vi "ELVIS III v1.0 DO Block Write.vi"(5 "Wait Until Done?":bool, 6 "DO FIFO Sample Rate (Hz)":dbl=1000.0 min=1000.0 max=8000000.0, 8 "error in (no error)":errorcluster, 9 "Data by Channel":bool[][](array[boolean]) caption="bool Value List", 10 "DO (N Samples) Channel List":T3, 11 "myRIO Ref In":T1) -> (0 "error out":errorcluster, 3 "myRIO Ref Out":T1)   [LabVIEW 2021]
uses:
  <vilib>/myRIO/Common/Instrument Driver Framework/myRIO v1.0/DO Block/typedefs/DO Block Channels List.ctl
  <vilib>/myRIO/Common/Instrument Driver Framework/myRIO v1.0/DO Block/typedefs/DO Block Channels Enum.ctl
  <vilib>/myRIO/Common/Instrument Driver Framework/Utilities/typedefs/myRIO v1.0 Reference.ctl
  <vilib>/myRIO/Common/Instrument Driver Framework/Utilities/typedefs/Generic FPGA Reference.ctl
  <vilib>/myRIO/Common/Instrument Driver Framework/ELVIS III v1.0/DO Block/typedefs/ELVIS III DO Block FPGA Reference.ctl
  <vilib>/myRIO/Common/Instrument Driver Framework/ELVIS III v1.0/DO Block/typedefs/ELVIS III DO Block Configuration.ctl
  <vilib>/myRIO/Common/Instrument Driver Framework/ELVIS III v1.0/DO Block/typedefs/ELVIS III DO Block Bank Data.ctl
  <vilib>/myRIO/Common/Instrument Driver Framework/myRIO v1.0/Resource Manager/vis/myRIO v1.0 Block Write Configuration.vi
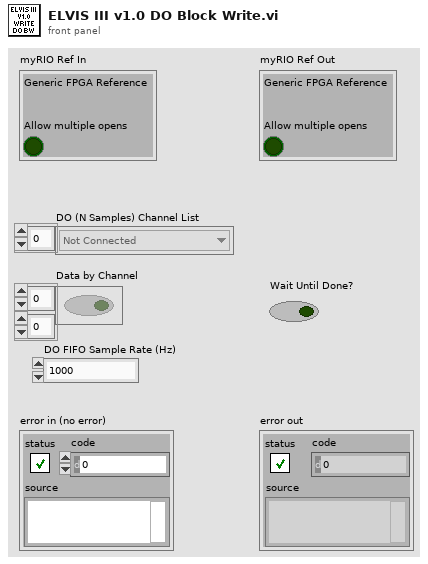
[diagram p1: front panel]
types:
  T1 = typedef "myRIO v1.0 Reference.ctl" = cluster{"Generic FPGA Reference":T2, "Allow multiple opens":bool}
  T2 = typedef "Generic FPGA Reference.ctl" = refnum<k20>
  T3 = typedef "DO Block Channels List.ctl" = T4[]
  T4 = typedef "DO Block Channels Enum.ctl" = enum16{"Not Connected", "A/DO0 (N Samples)", "A/DO1 (N Samples)", "A/DO2 (N Samples)", "A/DO3 (N Samples)", "A/DO4 (N Samples)", "A/DO5 (N Samples)", "A/DO6 (N Samples)", "A/DO7 (N Samples)", "A/DO8 (N Samples)", "A/DO9 (N Samples)", "A/DO10 (N Samples)", "A/DO11 (N Samples)", "A/DO12 (N Samples)", "A/DO13 (N Samples)", "A/DO14 (N Samples)", "A/DO15 (N Samples)", "A/DO16 (N Samples)", "A/DO17 (N Samples)", "A/DO18 (N Samples)", "A/DO19 (N Samples)", "B/DO0 (N Samples)", "B/DO1 (N Samples)", "B/DO2 (N Samples)", "B/DO3 (N Samples)", "B/DO4 (N Samples)", "B/DO5 (N Samples)", "B/DO6 (N Samples)", "B/DO7 (N Samples)", "B/DO8 (N Samples)", "B/DO9 (N Samples)", "B/DO10 (N Samples)", "B/DO11 (N Samples)", "B/DO12 (N Samples)", "B/DO13 (N Samples)", "B/DO14 (N Samples)", "B/DO15 (N Samples)", "B/DO16 (N Samples)", "B/DO17 (N Samples)", "B/DO18 (N Samples)", "B/DO19 (N Samples)"}
  T5 = typedef "ELVIS III DO Block FPGA Reference.ctl" = refnum<k20>
  T6 = typedef "ELVIS III DO Block Configuration.ctl" = cluster{"Wait Until Done?":bool, "DO FIFO Clock Divisor":u16, "Write Mode":u8, "DO (N Samples) Bank Data ":T7[]}
  T7 = typedef "ELVIS III DO Block Bank Data.ctl" = cluster{"Digital Data Reference":refnum<data-value>, "Channel  Bitmask":fxp<+,20,20>, "Semaphore":T8}
  T8 = typedef "Semaphore RefNum" = refnum<k1>
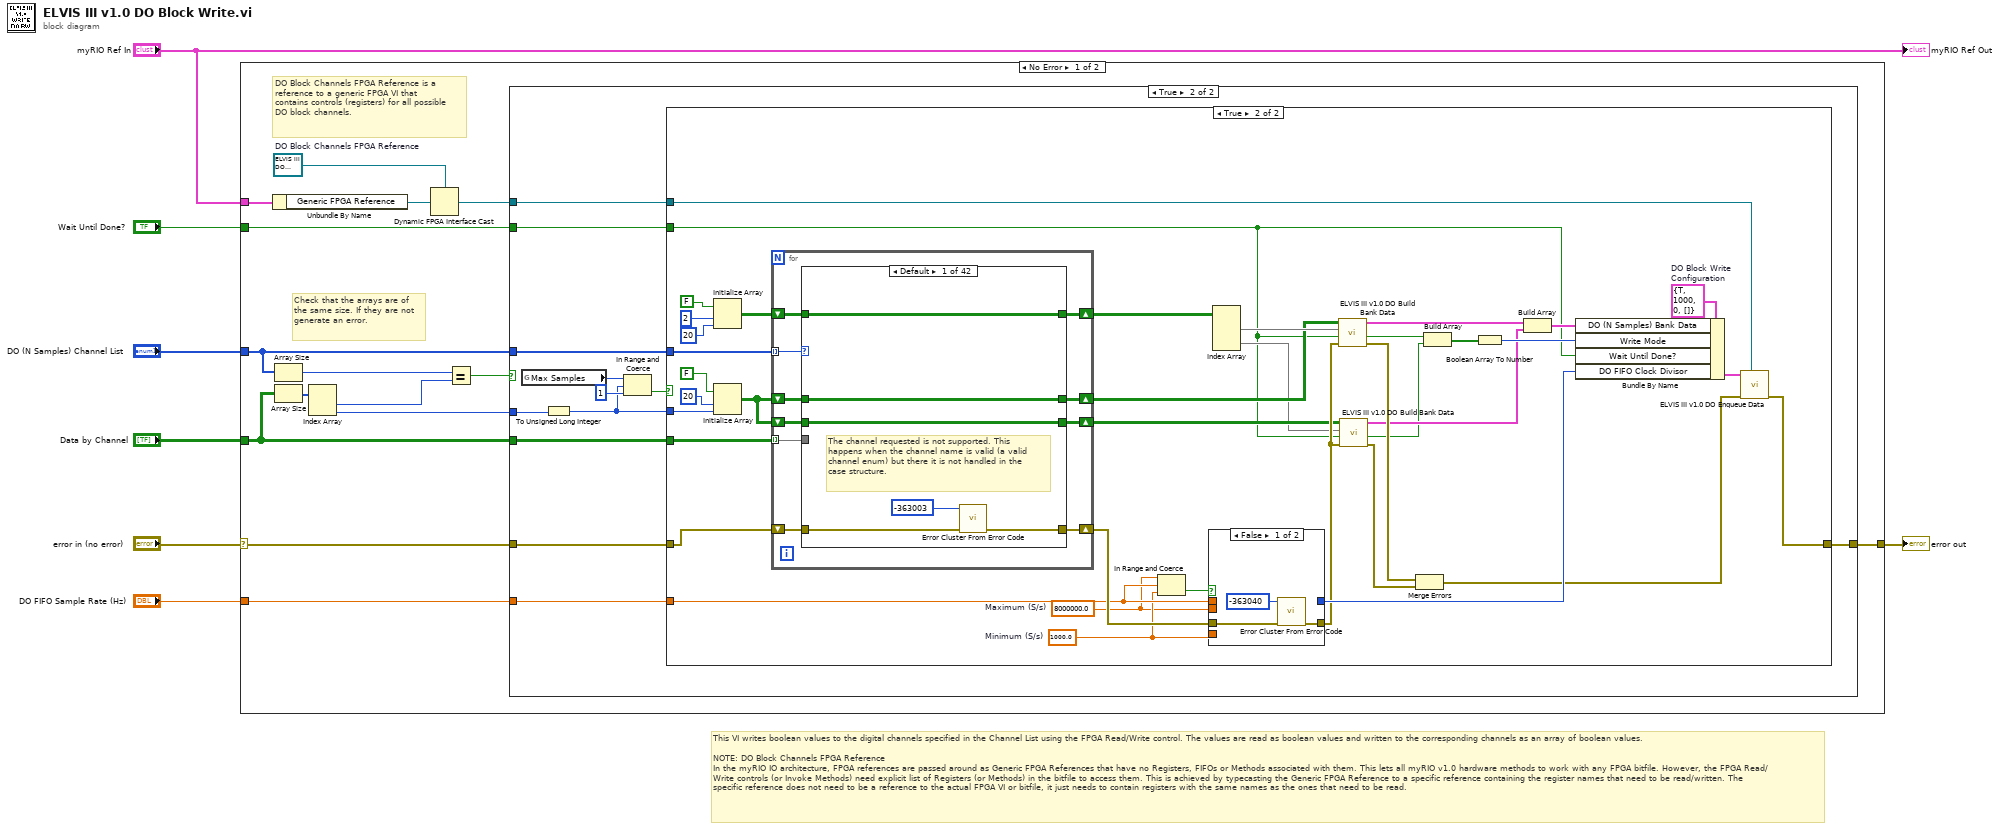
[diagram p0: block diagram]
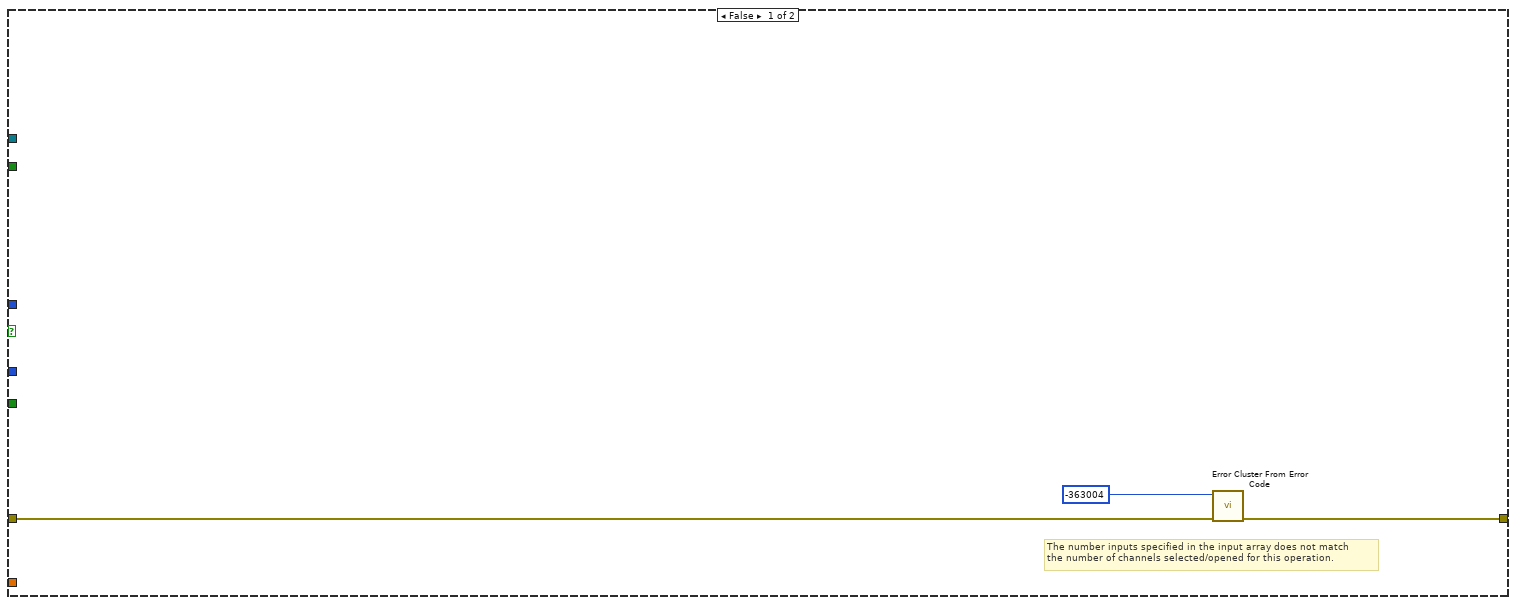
[diagram p2: hidden frame]
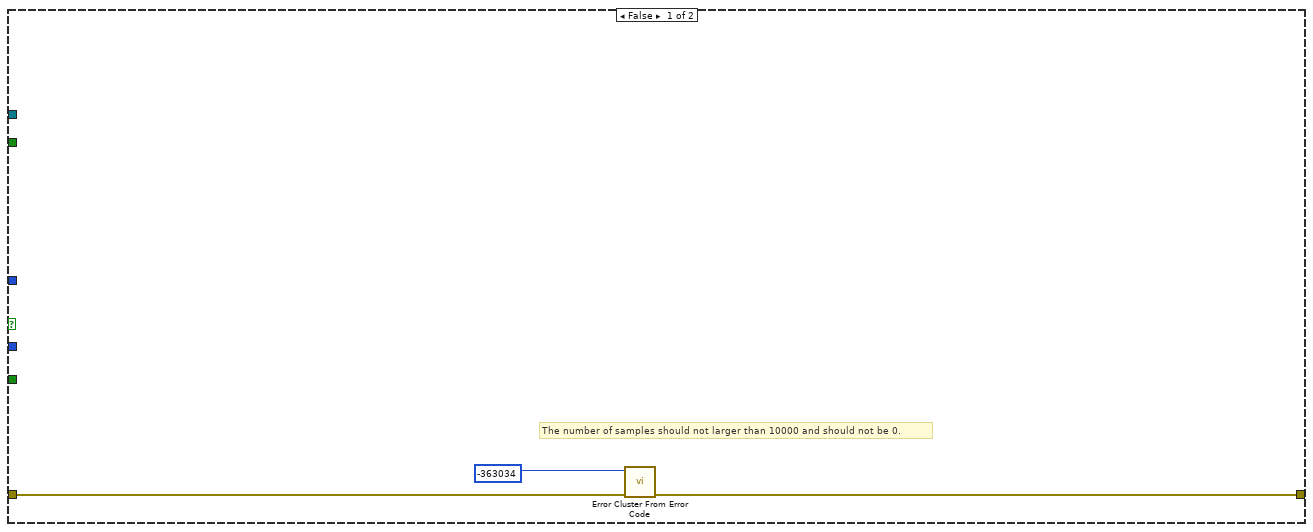
[diagram p3: hidden frame]
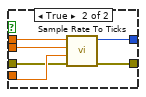
[diagram p4: hidden frame]
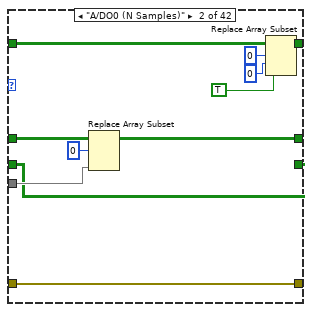
[diagram p5: hidden frame]
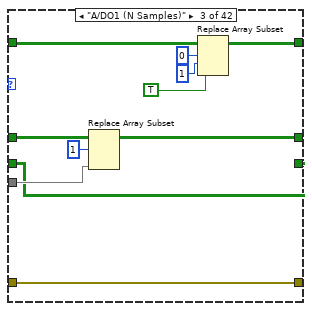
[diagram p6: hidden frame]
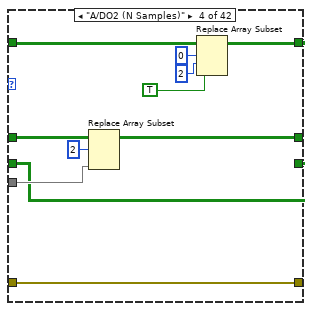
[diagram p7: hidden frame]
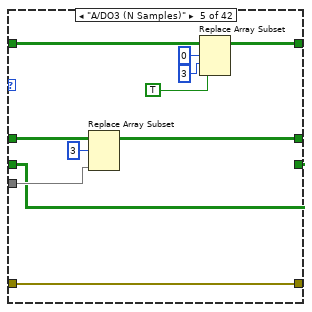
[diagram p8: hidden frame]
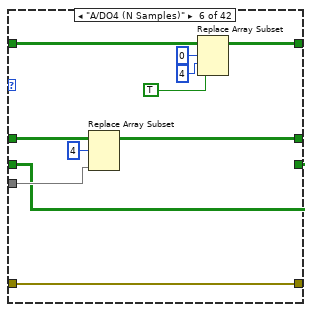
[diagram p9: hidden frame]
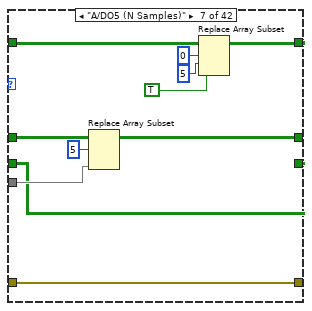
[diagram p10: hidden frame]
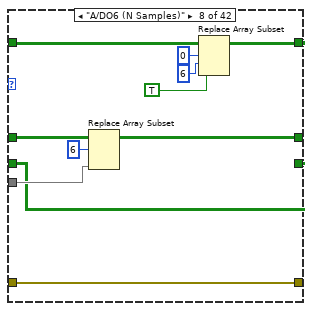
[diagram p11: hidden frame]
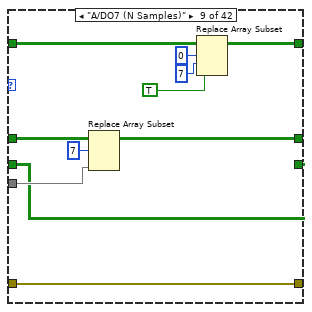
[diagram p12: hidden frame]
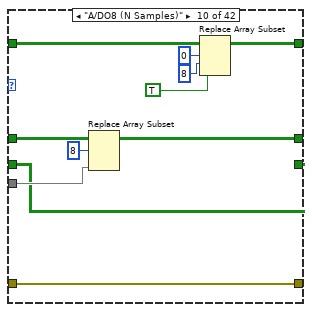
[diagram p13: hidden frame]
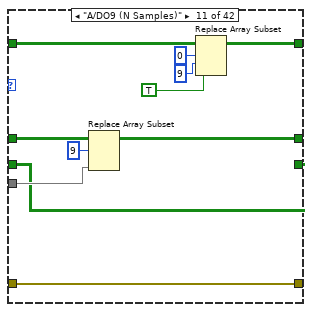
[diagram p14: hidden frame]
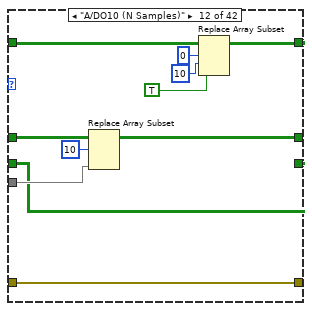
[diagram p15: hidden frame]
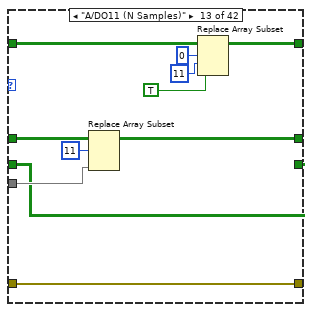
[diagram p16: hidden frame]
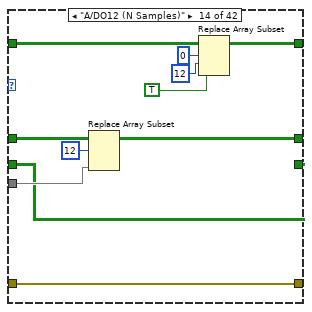
[diagram p17: hidden frame]
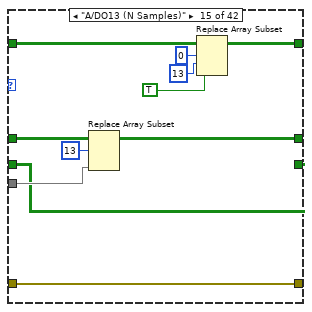
[diagram p18: hidden frame]
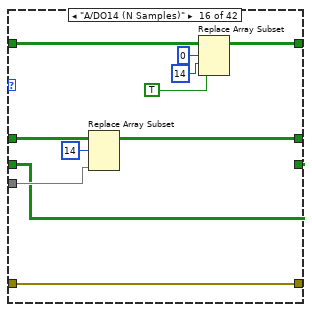
[diagram p19: hidden frame]
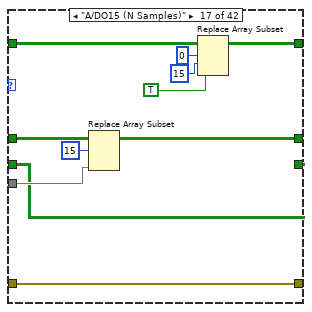
[diagram p20: hidden frame]
diagram:
  # "This VI writes boolean values to the digital channels specified in the Channel List using the FPGA Read/Write control. The values are read as boolean values and written to the corresponding channels as an array of boolean values. \n\nNOTE: DO Block Channels FPGA Reference\nIn the myRIO IO architecture, FPGA references are passed around as Generic FPGA References that have no Registers, FIFOs or Methods associated with them. This lets all myRIO v1.0 hardware methods to work with any FPGA bitfile. However, the FPGA Read/Write controls (or Invoke Methods) need explicit list of Registers (or Methods) in the bitfile to access them. This is achieved by typecasting the Generic FPGA Reference to a specific reference containing the register names that need to be read/written. The specific reference does not need to be a reference to the actual FPGA VI or bitfile, it just needs to contain registers with the same names as the ones that need to be read."
  n1 = case shown="No Error" "error in (no error)" {
    selector: "error in (no error)" -> [w8 w548]
    tunnel: "myRIO Ref In" -> [w22 _]
    tunnel: [w21 w548] -> w6
    tunnel: "DO (N Samples) Channel List" -> [w19 _]
    tunnel: "Data by Channel" -> [w18 _]
    tunnel: "DO FIFO Sample Rate (Hz)" -> [w9 _]
    tunnel: "Wait Until Done?" -> [w14 _]
    frame No Error {
      w13 = T5 refnum  # DO Block Channels FPGA Reference
      # "DO Block Channels FPGA Reference is a reference to a generic FPGA VI that contains controls (registers) for all possible DO block channels."
      # "Check that the arrays are of the same size. If they are not generate an error."
      n2 = Unbundle By Name(w22) -> ("Generic FPGA Reference"=w12:T2)
      n3 = Array Size(array=w19) -> (size(s)=w20:i32)
      n4 = Array Size(array=w18) -> (size(s)=w16:i32[])
      n5 = Index Array(array=w16) -> (element #1=w15:i32, element #2=w10:i32)  [unwired: 2 in]
      n6 = Dynamic FPGA Interface Cast(Session In=w13, Type=w12) -> (Session Out=w11:T5)
      n7 = Equal?(x=w20, y=w15) -> (x = y?=w17:bool)
      n8 = case shown="True" w17 {
        tunnel: w19 -> [_ w35]
        tunnel: w18 -> [_ w34]
        tunnel: w8 -> [w24 w37]
        tunnel: [w23 w36] -> w21
        tunnel: w9 -> [_ w27]
        tunnel: w14 -> [_ w26]
        tunnel: w11 -> [_ w28]
        tunnel: w10 -> [_ w33]
        frame False {
          # "The number inputs specified in the input array does not match\nthe number of channels selected/opened for this operation."
          n9 = call <vilib>:"Error Cluster From Error Code.vi"("error in (no error)"=w24, "error code (0)"=-363004) -> ("error out"=w23:errorcluster)  [unwired: 7 in]
        }
        frame True {
          n10 = global read "myRIO v1.0 Block Write Configuration.vi" "Max Samples"() -> (w31:u32)
          n11 = To Unsigned Long Integer(number=w33) -> (unsigned 32bit integer=w29:u32)
          n12 = In Range and Coerce(upper limit=w31, x=w29, lower limit=u32 1) -> (In Range?=w32:bool)  [unwired: 1 out]
          n13 = case shown="True" w32 {
            tunnel: w37 -> [w39 w78]
            tunnel: [w38 w66] -> w36
            tunnel: w35 -> [_ w77]
            tunnel: w34 -> [_ w76]
            tunnel: w29 -> [_ w72]
            tunnel: w28 -> [_ w67]
            tunnel: w27 -> [_ w44]
            tunnel: w26 -> [_ w50]
            frame False {
              # "The number of samples should not larger than 10000 and should not be 0."
              n14 = call <vilib>:"Error Cluster From Error Code.vi"("error in (no error)"=w39, "error code (0)"=-363034) -> ("error out"=w38:errorcluster)  [unwired: 7 in]
            }
            frame True {
              w62 = T6 {"Wait Until Done?"=TRUE, "DO FIFO Clock Divisor"=1000, "Write Mode"=0, "DO (N Samples) Bank Data "=[]}  # DO Block Write Configuration
              w43 = 1000.0  # Minimum (S/s)
              w42 = 8000000.0  # Maximum (S/s)
              n15 = Initialize Array(FALSE ("element"), 2 ("dimension size"), 20 ("dimension size")) -> (w69:bool[][])
              n16 = Initialize Array(FALSE, 20 ("dimension size"), w72) -> (w74:bool[][])
              n17 = for {
                shift-right: [w94] -> w65
                shift-left: w78 -> [w96]
                tunnel: w77 -> [w97] mode=indexing
                tunnel: w76 -> [w95] mode=indexing
                shift-right: [w88] -> w53
                shift-left: w74 -> [w93]
                shift-right: [w91] -> w52
                shift-left: w74 -> [w92]
                shift-right: [w89] -> w68
                shift-left: w69 -> [w90]
                n18 = case shown="Default" w97 {
                  tunnel: w96 -> [w102 w106 w120 w131 w142 w153 w164 w175 w186 w197 w208 w219 w230 w241 w252 w263 w274 w285 w296 w307 w318 w329 w340 w351 w362 w373 w384 w395 w406 w417 w428 w439 w450 w461 w472 w483 w494 w505 w516 w527 w538 w547]
                  tunnel: w95 -> [_ w112 w123 w134 w145 w156 w167 w178 w189 w200 w211 w222 w233 w244 w255 w266 w277 w288 w299 w310 w321 w333 w344 w355 w366 w377 w388 w399 w410 w421 w432 w443 w454 w465 w476 w487 w498 w509 w520 w531 w542 _]
                  tunnel: [w101 w106 w120 w131 w142 w153 w164 w175 w186 w197 w208 w219 w230 w241 w252 w263 w274 w285 w296 w307 w318 w329 w340 w351 w362 w373 w384 w395 w406 w417 w428 w439 w450 w461 w472 w483 w494 w505 w516 w527 w538 w547] -> w94
                  tunnel: w93 -> [w100 w114 w125 w136 w147 w158 w169 w180 w191 w202 w213 w224 w235 w246 w257 w268 w279 w290 w301 w312 w323 w330 w341 w352 w363 w374 w385 w396 w407 w418 w429 w440 w451 w462 w473 w484 w495 w506 w517 w528 w539 w546]
                  tunnel: [w100 w111 w122 w133 w144 w155 w166 w177 w188 w199 w210 w221 w232 w243 w254 w265 w276 w287 w298 w309 w320 w330 w341 w352 w363 w374 w385 w396 w407 w418 w429 w440 w451 w462 w473 w484 w495 w506 w517 w528 w539 w546] -> w88
                  tunnel: w92 -> [w99 w110 w121 w132 w143 w154 w165 w176 w187 w198 w209 w220 w231 w242 w253 w264 w275 w286 w297 w308 w319 w332 w343 w354 w365 w376 w387 w398 w409 w420 w431 w442 w453 w464 w475 w486 w497 w508 w519 w530 w541 w545]
                  tunnel: [w99 w110 w121 w132 w143 w154 w165 w176 w187 w198 w209 w220 w231 w242 w253 w264 w275 w286 w297 w308 w319 w331 w342 w353 w364 w375 w386 w397 w408 w419 w430 w441 w452 w463 w474 w485 w496 w507 w518 w529 w540 w545] -> w91
                  tunnel: w90 -> [w98 w109 w116 w127 w137 w148 w159 w170 w181 w192 w203 w214 w225 w236 w247 w258 w269 w280 w291 w302 w313 w324 w335 w346 w357 w368 w379 w390 w401 w412 w424 w434 w445 w456 w467 w478 w489 w500 w511 w522 w533 w544]
                  tunnel: [w98 w108 w115 w126 w138 w149 w160 w171 w182 w193 w204 w215 w226 w237 w248 w259 w270 w281 w292 w303 w314 w325 w336 w347 w358 w369 w380 w391 w402 w413 w423 w435 w446 w457 w468 w479 w490 w501 w512 w523 w534 w544] -> w89
                  frame Default {
                    # "The channel requested is not supported. This happens when the channel name is valid (a valid channel enum) but there it is not handled in the case structure."
                    n19 = call <vilib>:"Error Cluster From Error Code.vi"("error in (no error)"=w102, "error code (0)"=-363003) -> ("error out"=w101:errorcluster)  [unwired: 7 in]
                  }
                  frame "A/DO0 (N Samples)" {
                    n20 = Replace Array Subset(array=w114, new element=w112, index (row)=0) -> (w111:bool[][])  [unwired: 1 in]
                    n21 = Replace Array Subset(array=w109, new element=TRUE ("new element/subarray"), index (row)=0 ("index"), index (col)=0 ("disabled index (col)")) -> (w108:bool[][])
                  }
                  frame "A/DO1 (N Samples)" {
                    n22 = Replace Array Subset(array=w125, new element=w123, index (row)=1) -> (w122:bool[][])  [unwired: 1 in]
                    n23 = Replace Array Subset(array=w116, new element=TRUE ("new element/subarray"), index (row)=0 ("index"), index (col)=1 ("disabled index (col)")) -> (w115:bool[][])
                  }
                  frame "A/DO2 (N Samples)" {
                    n24 = Replace Array Subset(array=w136, new element=w134, index (row)=2) -> (w133:bool[][])  [unwired: 1 in]
                    n25 = Replace Array Subset(array=w127, new element=TRUE ("new element/subarray"), index (row)=0 ("index"), index (col)=2 ("disabled index (col)")) -> (w126:bool[][])
                  }
                  frame "A/DO3 (N Samples)" {
                    n26 = Replace Array Subset(array=w147, new element=w145, index (row)=3) -> (w144:bool[][])  [unwired: 1 in]
                    n27 = Replace Array Subset(array=w137, new element=TRUE ("new element/subarray"), index (row)=0 ("index"), index (col)=3 ("disabled index (col)")) -> (w138:bool[][])
                  }
                  frame "A/DO4 (N Samples)" {
                    n28 = Replace Array Subset(array=w158, new element=w156, index (row)=4) -> (w155:bool[][])  [unwired: 1 in]
                    n29 = Replace Array Subset(array=w148, new element=TRUE ("new element/subarray"), index (row)=0 ("index"), index (col)=4 ("disabled index (col)")) -> (w149:bool[][])
                  }
                  frame "A/DO5 (N Samples)" {
                    n30 = Replace Array Subset(array=w169, new element=w167, index (row)=5) -> (w166:bool[][])  [unwired: 1 in]
                    n31 = Replace Array Subset(array=w159, new element=TRUE ("new element/subarray"), index (row)=0 ("index"), index (col)=5 ("disabled index (col)")) -> (w160:bool[][])
                  }
                  frame "A/DO6 (N Samples)" {
                    n32 = Replace Array Subset(array=w180, new element=w178, index (row)=6) -> (w177:bool[][])  [unwired: 1 in]
                    n33 = Replace Array Subset(array=w170, new element=TRUE ("new element/subarray"), index (row)=0 ("index"), index (col)=6 ("disabled index (col)")) -> (w171:bool[][])
                  }
                  frame "A/DO7 (N Samples)" {
                    n34 = Replace Array Subset(array=w191, new element=w189, index (row)=7) -> (w188:bool[][])  [unwired: 1 in]
                    n35 = Replace Array Subset(array=w181, new element=TRUE ("new element/subarray"), index (row)=0 ("index"), index (col)=7 ("disabled index (col)")) -> (w182:bool[][])
                  }
                  frame "A/DO8 (N Samples)" {
                    n36 = Replace Array Subset(array=w202, new element=w200, index (row)=8) -> (w199:bool[][])  [unwired: 1 in]
                    n37 = Replace Array Subset(array=w192, new element=TRUE ("new element/subarray"), index (row)=0 ("index"), index (col)=8 ("disabled index (col)")) -> (w193:bool[][])
                  }
                  frame "A/DO9 (N Samples)" {
                    n38 = Replace Array Subset(array=w213, new element=w211, index (row)=9) -> (w210:bool[][])  [unwired: 1 in]
                    n39 = Replace Array Subset(array=w203, new element=TRUE ("new element/subarray"), index (row)=0 ("index"), index (col)=9 ("disabled index (col)")) -> (w204:bool[][])
                  }
                  frame "A/DO10 (N Samples)" {
                    n40 = Replace Array Subset(array=w224, new element=w222, index (row)=10) -> (w221:bool[][])  [unwired: 1 in]
                    n41 = Replace Array Subset(array=w214, new element=TRUE ("new element/subarray"), index (row)=0 ("index"), index (col)=10 ("disabled index (col)")) -> (w215:bool[][])
                  }
                  frame "A/DO11 (N Samples)" {
                    n42 = Replace Array Subset(array=w235, new element=w233, index (row)=11) -> (w232:bool[][])  [unwired: 1 in]
                    n43 = Replace Array Subset(array=w225, new element=TRUE ("new element/subarray"), index (row)=0 ("index"), index (col)=11 ("disabled index (col)")) -> (w226:bool[][])
                  }
                  frame "A/DO12 (N Samples)" {
                    n44 = Replace Array Subset(array=w246, new element=w244, index (row)=12) -> (w243:bool[][])  [unwired: 1 in]
                    n45 = Replace Array Subset(array=w236, new element=TRUE ("new element/subarray"), index (row)=0 ("index"), index (col)=12 ("disabled index (col)")) -> (w237:bool[][])
                  }
                  frame "A/DO13 (N Samples)" {
                    n46 = Replace Array Subset(array=w257, new element=w255, index (row)=13) -> (w254:bool[][])  [unwired: 1 in]
                    n47 = Replace Array Subset(array=w247, new element=TRUE ("new element/subarray"), index (row)=0 ("index"), index (col)=13 ("disabled index (col)")) -> (w248:bool[][])
                  }
                  frame "A/DO14 (N Samples)" {
                    n48 = Replace Array Subset(array=w268, new element=w266, index (row)=14) -> (w265:bool[][])  [unwired: 1 in]
                    n49 = Replace Array Subset(array=w258, new element=TRUE ("new element/subarray"), index (row)=0 ("index"), index (col)=14 ("disabled index (col)")) -> (w259:bool[][])
                  }
                  frame "A/DO15 (N Samples)" {
                    n50 = Replace Array Subset(array=w279, new element=w277, index (row)=15) -> (w276:bool[][])  [unwired: 1 in]
                    n51 = Replace Array Subset(array=w269, new element=TRUE ("new element/subarray"), index (row)=0 ("index"), index (col)=15 ("disabled index (col)")) -> (w270:bool[][])
                  }
                  frame "A/DO16 (N Samples)" {
                    n52 = Replace Array Subset(array=w290, new element=w288, index (row)=16) -> (w287:bool[][])  [unwired: 1 in]
                    n53 = Replace Array Subset(array=w280, new element=TRUE ("new element/subarray"), index (row)=0 ("index"), index (col)=16 ("disabled index (col)")) -> (w281:bool[][])
                  }
                  frame "A/DO17 (N Samples)" {
                    n54 = Replace Array Subset(array=w301, new element=w299, index (row)=17) -> (w298:bool[][])  [unwired: 1 in]
                    n55 = Replace Array Subset(array=w291, new element=TRUE ("new element/subarray"), index (row)=0 ("index"), index (col)=17 ("disabled index (col)")) -> (w292:bool[][])
                  }
                  frame "A/DO18 (N Samples)" {
                    n56 = Replace Array Subset(array=w312, new element=w310, index (row)=18) -> (w309:bool[][])  [unwired: 1 in]
                    n57 = Replace Array Subset(array=w302, new element=TRUE ("new element/subarray"), index (row)=0 ("index"), index (col)=18 ("disabled index (col)")) -> (w303:bool[][])
                  }
                  frame "A/DO19 (N Samples)" {
                    n58 = Replace Array Subset(array=w323, new element=w321, index (row)=19) -> (w320:bool[][])  [unwired: 1 in]
                    n59 = Replace Array Subset(array=w313, new element=TRUE ("new element/subarray"), index (row)=0 ("index"), index (col)=19 ("disabled index (col)")) -> (w314:bool[][])
                  }
                  frame "B/DO0 (N Samples)" {
                    n60 = Replace Array Subset(array=w332, new element=w333, index (row)=0) -> (w331:bool[][])  [unwired: 1 in]
                    n61 = Replace Array Subset(array=w324, new element=TRUE ("new element/subarray"), index (row)=1 ("index"), index (col)=0 ("disabled index (col)")) -> (w325:bool[][])
                  }
                  frame "B/DO1 (N Samples)" {
                    n62 = Replace Array Subset(array=w343, new element=w344, index (row)=1) -> (w342:bool[][])  [unwired: 1 in]
                    n63 = Replace Array Subset(array=w335, new element=TRUE ("new element/subarray"), index (row)=1 ("index"), index (col)=1 ("disabled index (col)")) -> (w336:bool[][])
                  }
                  frame "B/DO2 (N Samples)" {
                    n64 = Replace Array Subset(array=w354, new element=w355, index (row)=2) -> (w353:bool[][])  [unwired: 1 in]
                    n65 = Replace Array Subset(array=w346, new element=TRUE ("new element/subarray"), index (row)=1 ("index"), index (col)=2 ("disabled index (col)")) -> (w347:bool[][])
                  }
                  frame "B/DO3 (N Samples)" {
                    n66 = Replace Array Subset(array=w365, new element=w366, index (row)=3) -> (w364:bool[][])  [unwired: 1 in]
                    n67 = Replace Array Subset(array=w357, new element=TRUE ("new element/subarray"), index (row)=1 ("index"), index (col)=3 ("disabled index (col)")) -> (w358:bool[][])
                  }
                  frame "B/DO4 (N Samples)" {
                    n68 = Replace Array Subset(array=w376, new element=w377, index (row)=4) -> (w375:bool[][])  [unwired: 1 in]
                    n69 = Replace Array Subset(array=w368, new element=TRUE ("new element/subarray"), index (row)=1 ("index"), index (col)=4 ("disabled index (col)")) -> (w369:bool[][])
                  }
                  frame "B/DO5 (N Samples)" {
                    n70 = Replace Array Subset(array=w387, new element=w388, index (row)=5) -> (w386:bool[][])  [unwired: 1 in]
                    n71 = Replace Array Subset(array=w379, new element=TRUE ("new element/subarray"), index (row)=1 ("index"), index (col)=5 ("disabled index (col)")) -> (w380:bool[][])
                  }
                  frame "B/DO6 (N Samples)" {
                    n72 = Replace Array Subset(array=w398, new element=w399, index (row)=6) -> (w397:bool[][])  [unwired: 1 in]
                    n73 = Replace Array Subset(array=w390, new element=TRUE ("new element/subarray"), index (row)=1 ("index"), index (col)=6 ("disabled index (col)")) -> (w391:bool[][])
                  }
                  frame "B/DO7 (N Samples)" {
                    n74 = Replace Array Subset(array=w409, new element=w410, index (row)=7) -> (w408:bool[][])  [unwired: 1 in]
                    n75 = Replace Array Subset(array=w401, new element=TRUE ("new element/subarray"), index (row)=1 ("index"), index (col)=7 ("disabled index (col)")) -> (w402:bool[][])
                  }
                  frame "B/DO8 (N Samples)" {
                    n76 = Replace Array Subset(array=w420, new element=w421, index (row)=8) -> (w419:bool[][])  [unwired: 1 in]
                    n77 = Replace Array Subset(array=w412, new element=TRUE ("new element/subarray"), index (row)=1 ("index"), index (col)=8 ("disabled index (col)")) -> (w413:bool[][])
                  }
                  frame "B/DO9 (N Samples)" {
                    n78 = Replace Array Subset(array=w431, new element=w432, index (row)=9) -> (w430:bool[][])  [unwired: 1 in]
                    n79 = Replace Array Subset(array=w424, new element=TRUE ("new element/subarray"), index (row)=1 ("index"), index (col)=9 ("disabled index (col)")) -> (w423:bool[][])
                  }
                  frame "B/DO10 (N Samples)" {
                    n80 = Replace Array Subset(array=w442, new element=w443, index (row)=10) -> (w441:bool[][])  [unwired: 1 in]
                    n81 = Replace Array Subset(array=w434, new element=TRUE ("new element/subarray"), index (row)=1 ("index"), index (col)=10 ("disabled index (col)")) -> (w435:bool[][])
                  }
                  frame "B/DO11 (N Samples)" {
                    n82 = Replace Array Subset(array=w453, new element=w454, index (row)=11) -> (w452:bool[][])  [unwired: 1 in]
                    n83 = Replace Array Subset(array=w445, new element=TRUE ("new element/subarray"), index (row)=1 ("index"), index (col)=11 ("disabled index (col)")) -> (w446:bool[][])
                  }
                  frame "B/DO12 (N Samples)" {
                    n84 = Replace Array Subset(array=w464, new element=w465, index (row)=12) -> (w463:bool[][])  [unwired: 1 in]
                    n85 = Replace Array Subset(array=w456, new element=TRUE ("new element/subarray"), index (row)=1 ("index"), index (col)=12 ("disabled index (col)")) -> (w457:bool[][])
                  }
                  frame "B/DO13 (N Samples)" {
                    n86 = Replace Array Subset(array=w475, new element=w476, index (row)=13) -> (w474:bool[][])  [unwired: 1 in]
                    n87 = Replace Array Subset(array=w467, new element=TRUE ("new element/subarray"), index (row)=1 ("index"), index (col)=13 ("disabled index (col)")) -> (w468:bool[][])
                  }
                  frame "B/DO14 (N Samples)" {
                    n88 = Replace Array Subset(array=w486, new element=w487, index (row)=14) -> (w485:bool[][])  [unwired: 1 in]
                    n89 = Replace Array Subset(array=w478, new element=TRUE ("new element/subarray"), index (row)=1 ("index"), index (col)=14 ("disabled index (col)")) -> (w479:bool[][])
                  }
                  frame "B/DO15 (N Samples)" {
                    n90 = Replace Array Subset(array=w497, new element=w498, index (row)=15) -> (w496:bool[][])  [unwired: 1 in]
                    n91 = Replace Array Subset(array=w489, new element=TRUE ("new element/subarray"), index (row)=1 ("index"), index (col)=15 ("disabled index (col)")) -> (w490:bool[][])
                  }
                  frame "B/DO16 (N Samples)" {
                    n92 = Replace Array Subset(array=w508, new element=w509, index (row)=16) -> (w507:bool[][])  [unwired: 1 in]
                    n93 = Replace Array Subset(array=w500, new element=TRUE ("new element/subarray"), index (row)=1 ("index"), index (col)=16 ("disabled index (col)")) -> (w501:bool[][])
                  }
                  frame "B/DO17 (N Samples)" {
                    n94 = Replace Array Subset(array=w519, new element=w520, index (row)=17) -> (w518:bool[][])  [unwired: 1 in]
                    n95 = Replace Array Subset(array=w511, new element=TRUE ("new element/subarray"), index (row)=1 ("index"), index (col)=17 ("disabled index (col)")) -> (w512:bool[][])
                  }
                  frame "B/DO18 (N Samples)" {
                    n96 = Replace Array Subset(array=w530, new element=w531, index (row)=18) -> (w529:bool[][])  [unwired: 1 in]
                    n97 = Replace Array Subset(array=w522, new element=TRUE ("new element/subarray"), index (row)=1 ("index"), index (col)=18 ("disabled index (col)")) -> (w523:bool[][])
                  }
                  frame "B/DO19 (N Samples)" {
                    n98 = Replace Array Subset(array=w541, new element=w542, index (row)=19) -> (w540:bool[][])  [unwired: 1 in]
                    n99 = Replace Array Subset(array=w533, new element=TRUE ("new element/subarray"), index (row)=1 ("index"), index (col)=19 ("disabled index (col)")) -> (w534:bool[][])
                  }
                  frame "Not Connected" {
                  }
                }
              }
              n100 = In Range and Coerce(upper limit=w42, x=w44, lower limit=w43) -> (In Range?=w41:bool)  [unwired: 1 out]
              n101 = case shown="False" w41 {
                tunnel: w42 -> [_ w87]
                tunnel: w43 -> [_ w86]
                tunnel: w44 -> [_ w85]
                tunnel: w65 -> [w79 w84]
                tunnel: [_ w83] -> w64
                tunnel: [w80 w82] -> w58
                frame False {
                  n102 = call <vilib>:"Error Cluster From Error Code.vi"("error in (no error)"=w79, "error code (0)"=-363040) -> ("error out"=w80:errorcluster)  [unwired: 7 in]
                }
                frame True {
                  n103 = call <vilib>:"Sample Rate To Ticks.vi"("error in (no error)"=w84, "Minimum (S/s)"=w86, "Maximum (S/s)"=w87, "Sample Rate (S/s)"=w85) -> ("error out"=w82:errorcluster, "Count (tick/s)"=w83:u32)  [unwired: 5 in, 1 out]
                }
              }
              n104 = Index Array(array=w68) -> (element #1=w54:bool[], element #2=w51:bool[])  [unwired: 4 in]
              n105 = call <vilib>:"ELVIS III v1.0 DO Build Bank Data.vi"("error in (no error)"=w58, "Wait Until Done?"=w50, "Channel Bitmask"=w54, "Bank Data"=w53) -> ("error out"=w57:errorcluster, "Channel Selected?"=w47:bool, "Bank Data"=w49:T7)  [unwired: 5 in]
              n106 = call <vilib>:"ELVIS III v1.0 DO Build Bank Data.vi"("error in (no error)"=w58, "Wait Until Done?"=w50, "Channel Bitmask"=w51, "Bank Data"=w52) -> ("error out"=w56:errorcluster, "Channel Selected?"=w46:bool, "Bank Data"=w48:T7)  [unwired: 5 in]
              n107 = Merge Errors(w57, w56) -> (w55:errorcluster)
              n108 = Build Array(w47, w46) -> (w45:bool[])
              n109 = Boolean Array To Number(Boolean array=w45) -> (number=w59:u8)
              n110 = Build Array(w49, w48) -> (w60:T7[])
              n111 = Bundle By Name(cluster=w62, "DO (N Samples) Bank Data"=w60, "Write Mode"=w59, "Wait Until Done?"=w50, "DO FIFO Clock Divisor"=w64) -> (w61:T6)
              n112 = call <vilib>:"ELVIS III v1.0 DO Enqueue Data.vi"("DO Block Channels FPGA Reference"=w67, "error in (no error)"=w55, "DO Block Write Configuration"=w61) -> ("error out"=w66:errorcluster)  [unwired: 8 in]
            }
          }
        }
      }
    }
    frame Error {
    }
  }
  "error out" <- w6
  "myRIO Ref Out" <- "myRIO Ref In"
